vi "Generate String Buffer.vi"(1 "buffer size":i32) -> (0 "string buffer":string)   [LabVIEW 2020, in "MacroAssert.lvlib" / "Win Util New.lvlib"]
uses:
  Win Util New.lvlib
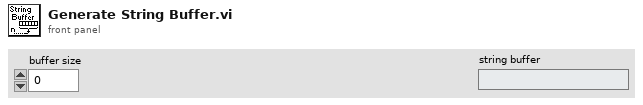
[diagram p1: front panel]
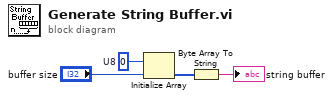
[diagram p0: block diagram]
diagram:
  w3 = u8 0  # U8
  n1 = Initialize Array(w3, "buffer size") -> (w2:u8[])
  n2 = Byte Array To String(unsigned byte array=w2) -> (string=→"string buffer":string)
